vi "QCA - DUT Generate Rx Command Dll.vi"(8 "Rx_Chan In":i32, 9 "Test_Index_r":i32, 10 "numPackets":i32=100, 11 "Rx_TV_Path":string) -> (0 "Freq_MHz":i32, 1 "Num_TestIndex":i32, 2 "SetRate_r":i32[](array[numeric]), 3 "RxCommand":string)   [LabVIEW 2011]
uses:
  TV/RW/Includes/WLAN - TV - RW - INC - RxTestParameters.ctl
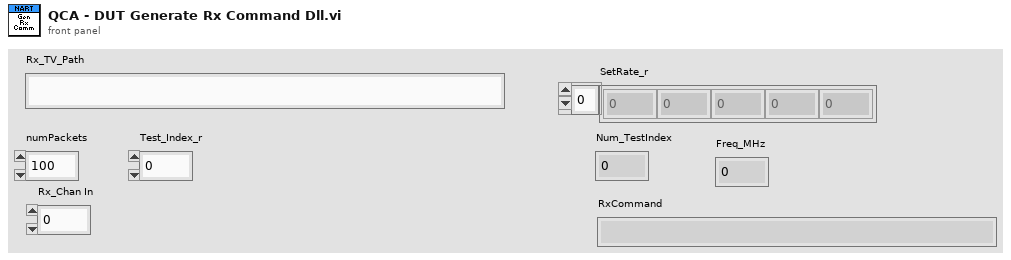
[diagram p1: front panel]
types:
  T1 = typedef "WLAN - TV - RW - INC - RxTestParameters.ctl" = cluster{"wfm Size in msec":i32, "actual headroom (dB)":dbl, "Size in Samples":i32[], "40M?":bool, "Standard ":i32, "wfm size sec (dbl)":dbl, "dt":dbl, "Channel Bandwidth (Hz)":dbl, "Payload Data Length (bytes)":i32, "80211n PLCP Frame Format":i32, "DSSS Data Rate (Mbps)":i32, "OFDM Data Rate (Mbps)":i32, "MCS Index":i32, "Fc(Hz)":dbl, "#Packets":i32}
  T2 = typedef "WLAN - TV - RW - INC - Rx_PER_Sweep_Settings.ctl" = cluster{"Wfm_Index":i32, "Power Level Settings":cluster{"Stop Power Level(dBm)":dbl, "Start Power Level(dBm)":dbl, "Step Size":dbl}, "Carrier Frequency(Hz)":dbl, "# Freq Points":i32}
  T3 = typedef "WLAN - TV - RW - INC - Rx_PER_Wfm_Settings.ctl" = cluster{"Standard":i32, "Channel Bandwidth (Hz)":dbl, "Idle Interval (s)":dbl, "MCS Index":i32, "80211n PLCP Frame Format":i32, "Payload Data Length (bytes)":i32, "OFDM Data Rate (Mbps)":i32, "DSSS Data Rate (Mbps)":i32, "Wfm_Index":i32}
  T4 = typedef "Data Rates.ctl" = string
  T5 = cluster{"Frequency, MHz":u32, "Data Rate":T4, "Packet Count":i32, "RX Mac Address":string, "TX Mac Address":string, "BS Mac Address":string, "Packet Length":u32, "Broadcast":bool}
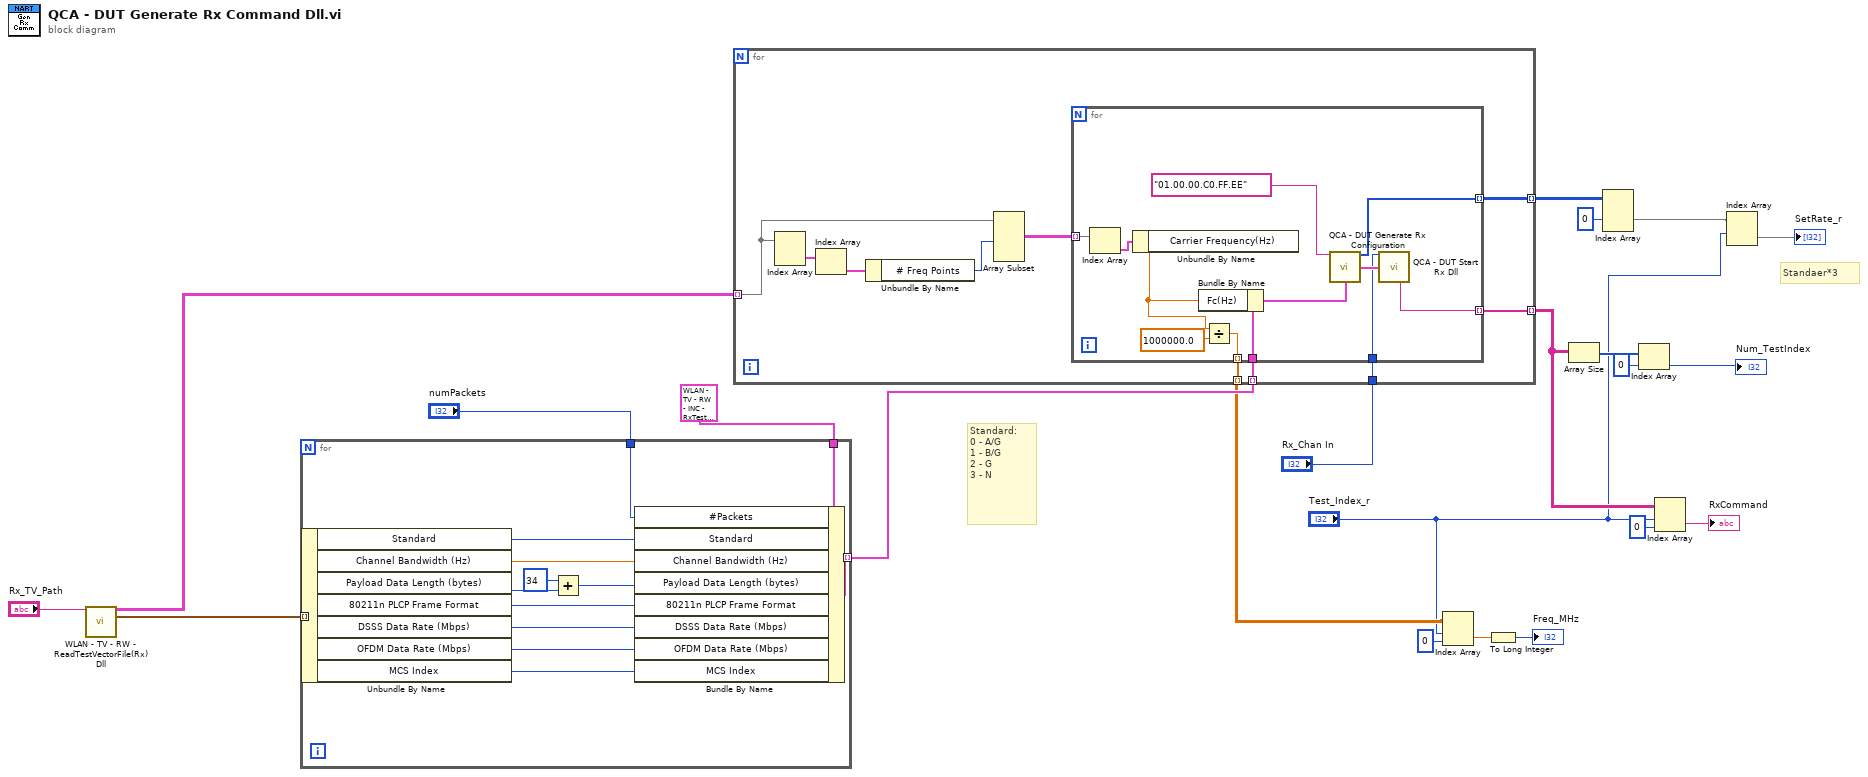
[diagram p0: block diagram]
diagram:
  # "Standaer*3"
  # "Standard:\n0 - A/G\n1 - B/G\n2 - G\n3 - N"
  n1 = call "WLAN - TV - RW - ReadTestVectorFile(Rx) Dll.vi"("Rx_TV_Path"="Rx_TV_Path") -> ("PER Sweep Settings(Wfm * FreQ * Pwr)"=w19:T2[][][], "Waveform Generation Settings"=w20:T3[])  [unwired: 11 in, 2 out]
  n2 = for {
    tunnel: T1 {"wfm Size in msec"=0, "actual headroom (dB)"=0.0, "Size in Samples"=[], "40M?"=FALSE, "Standard "=0, "wfm size sec (dbl)"=0.0, "dt"=0.0, "Channel Bandwidth (Hz)"=0.0, "Payload Data Length (bytes)"=0, "80211n PLCP Frame Format"=0, "DSSS Data Rate (Mbps)"=0, "OFDM Data Rate (Mbps)"=0, "MCS Index"=0, "Fc(Hz)"=0.0, "#Packets"=0} ("Cluster") -> [w35]
    tunnel: [w34] -> w18 mode=indexing
    tunnel: w20 -> [w33] mode=indexing
    tunnel: "numPackets" -> [w24]
    n3 = Unbundle By Name(w33) -> ("Standard"=w23:i32, "Channel Bandwidth (Hz)"=w32:dbl, "Payload Data Length (bytes)"=w31:i32, "80211n PLCP Frame Format"=w30:i32, "DSSS Data Rate (Mbps)"=w29:i32, "OFDM Data Rate (Mbps)"=w28:i32, "MCS Index"=w27:i32)
    n4 = Add(x=34, y=w31) -> (x+y=w26:i32)
    n5 = Bundle By Name(cluster=w35, "#Packets"=w24, "Standard"=w23, "Channel Bandwidth (Hz)"=w32, "Payload Data Length (bytes)"=w26, "80211n PLCP Frame Format"=w30, "DSSS Data Rate (Mbps)"=w29, "OFDM Data Rate (Mbps)"=w28, "MCS Index"=w27) -> (w34:T1)
  }
  n6 = for {
    tunnel: w19 -> [w42] mode=indexing
    tunnel: w18 -> [w40] mode=indexing
    tunnel: [w39] -> w11 mode=indexing
    tunnel: [w38] -> w6 mode=indexing
    tunnel: [w37] -> w16 mode=indexing
    tunnel: "Rx_Chan In" -> [w36]
    n7 = Index Array(array=w42) -> (element=w43:T2[])  [unwired: 2 in]
    n8 = Index Array(array=w43) -> (element=w44:T2)  [unwired: 1 in]
    n9 = Unbundle By Name(w44) -> ("# Freq Points"=w45:i32)
    n10 = Array Subset(array=w42, length (row)=w45) -> (w41:T2[][])  [unwired: 3 in]
    n11 = for {
      tunnel: w41 -> [w57] mode=indexing
      tunnel: w40 -> [w55]
      tunnel: [w52] -> w39 mode=indexing
      tunnel: [w47] -> w38 mode=indexing
      tunnel: [w50] -> w37 mode=indexing
      tunnel: w36 -> [w46]
      n12 = Index Array(array=w57) -> (element=w56:T2)  [unwired: 1 in]
      n13 = Unbundle By Name(w56) -> ("Carrier Frequency(Hz)"=w48:dbl)
      n14 = Bundle By Name(cluster=w55, "Fc(Hz)"=w48) -> (w54:T1)
      n15 = Divide(x=w48, y=1000000.0 ("x")) -> (x/y=w47:dbl)
      n16 = call "QCA - DUT Generate Rx Configuration.vi"("Mac Address"="01.00.00.C0.FF.EE", "Rx_Test Parameters"=w54) -> ("RateSet_r"=w50:i32[], "Rx Configuration"=w53:T5)  [unwired: 11 in, 1 out]
      n17 = call "QCA - DUT Start Rx Dll.vi"("Rx_Chan"=w46, "Receive Config"=w53) -> ("Command Sent"=w52:string)  [unwired: 12 in, 1 out]
    }
  }
  n18 = Index Array(array=w6, index (row)="Test_Index_r", index (col)=0 ("disabled index (col)")) -> (element=w3:dbl)
  n19 = To Long Integer(number=w3) -> (32bit integer=→"Freq_MHz":i32)
  n20 = Array Size(array=w11) -> (size(s)=w14:i32[])
  n21 = Index Array(array=w16, index (dim 1)=0 ("disabled index (row)")) -> (element=w8:i32[][])  [unwired: 2 in]
  n22 = Index Array(array=w14, index=0) -> (element=→"Num_TestIndex":i32)
  n23 = Index Array(array=w11, index (row)="Test_Index_r", index (col)=0 ("disabled index (col)")) -> (element=→"RxCommand":string)
  n24 = Index Array(array=w8, index (row)="Test_Index_r") -> (element=→"SetRate_r":i32[])  [unwired: 1 in]
